vi "Data Write.vi"(4 "File Type":T1, 6 "Append Index":i32, 8 "error in (no error)":errorcluster, 9 "Notes":string, 10 "Data (Dictionary)":T2[](array[typedef]), 11 "path":path) -> (0 "error out":errorcluster, 3 "path out":path)   [LabVIEW 2019, in "Data.lvclass"]
uses:
  Data.lvclass
  Typedefs/Operation--enum.ctl
  Typedefs/Dictionary--cluster.ctl
  Typedefs/File Type--enum.ctl
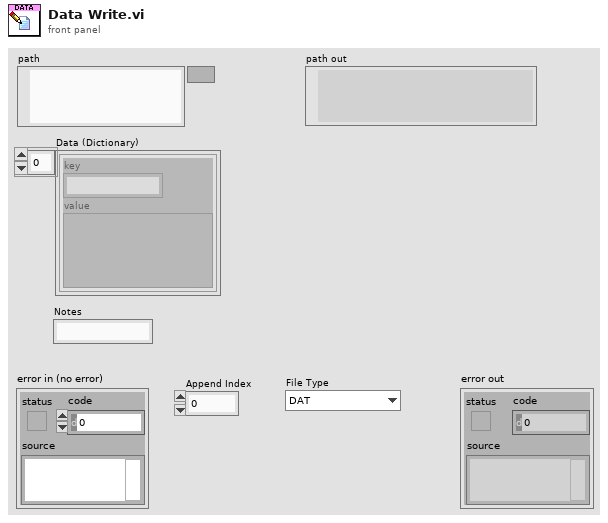
[diagram p1: front panel]
types:
  T1 = typedef "Data.lvclass/File Type--enum.ctl" = enum16{"DAT", "ITX", "TDMS", "VI"}
  T2 = typedef "Data.lvclass/Dictionary--cluster.ctl" = cluster{"key":string, "value":variant}
  T3 = typedef "Data.lvclass/Operation--enum.ctl" = enum16{"Read", "Write", "Write + Append"}
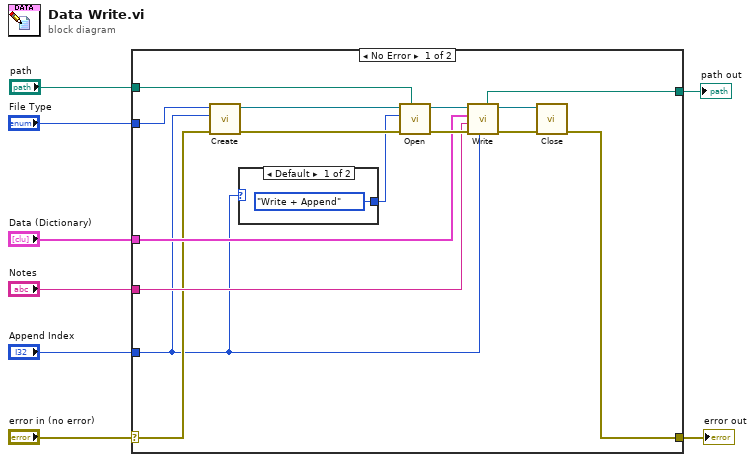
[diagram p0: block diagram]
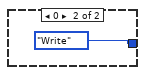
[diagram p2: hidden frame]
diagram:
  n1 = case shown="No Error" "error in (no error)" {
    selector: "error in (no error)" -> [w12 w27]
    tunnel: [w11 w27] -> w7
    tunnel: "path" -> [w15 w26]
    tunnel: "Data (Dictionary)" -> [w19 _]
    tunnel: "Notes" -> [w18 _]
    tunnel: "File Type" -> [w13 _]
    tunnel: "Append Index" -> [w9 _]
    tunnel: [w14 w26] -> w2
    frame No Error {
      n2 = call "Create.vi"("error in (no error)"=w12, "Append Index (-1)"=w9, "File Type"=w13) -> ("error out"=w23:errorcluster, "Data out"=w22:refnum<class "Data.lvclass">)  [unwired: 7 in]
      n3 = case shown="Default" w9 {
        tunnel: [Operation--enum."Write + Append" ("Operation") Operation--enum."Write" ("Operation")] -> w10
        frame Default {
        }
        frame 0 {
        }
      }
      n4 = call-dynamic "Open.vi"("Path"=w15, "error in (no error)"=w23, "Operation"=w10, "Data in"=w22) -> ("error out"=w20:errorcluster, "Data out"=w21:refnum<class "Data.lvclass">)  [unwired: 6 in]
      n5 = call-dynamic "Write.vi"("Append Index"=w9, "error in (no error)"=w20, "Notes"=w18, "Data (Dictionary)"=w19, "Data in"=w21) -> ("error out"=w17:errorcluster, "Data out"=w16:refnum<class "Data.lvclass">, "Path out"=w14:path)  [unwired: 4 in]
      n6 = call-dynamic "Close.vi"("error in (no error)"=w17, "Data in"=w16) -> ("error out"=w11:errorcluster)  [unwired: 8 in, 1 out]
    }
    frame Error {
    }
  }
  "error out" <- w7
  "path out" <- w2
